vi "Get Template Path.vi"(11 "Concrete Message Scripter in":refnum<class "Concrete Message Scripter.lvclass">) -> (2 "Template Path":path)   [LabVIEW 2020, in "Message Maker.lvlib" / "Concrete Message Scripter.lvclass"]
uses:
  Concrete Message Scripter.lvclass
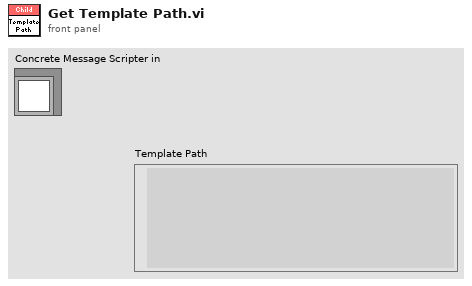
[diagram p1: front panel]
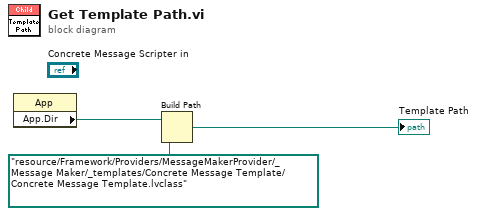
[diagram p0: block diagram]
diagram:
  n1 = property class="App"() -> ("App.Dir"=w1:path)  [unwired: 2 in, 2 out]
  n2 = Build Path(base path=w1, name or relative path=path "resource/Framework/Providers/MessageMakerProvider/_Message Maker/_templates/Concrete Message Template/Concrete Message Template.lvclass" ("class path")) -> (appended path=→"Template Path":path)
